vi "Shared Variable RT Driver VI.vi"(7 "Operation":T1, 11 "Device Reference in":T2 format="%.0x") -> (0 "Error Code":i32)   [LabVIEW 2015, in "Shared Variable Custom Device.lvlib"]
uses:
  Shared Variable Custom Device.lvlib
  <vilib>/NI Veristand/Custom Device API/Custom Device Item Ref.ctl
  <vilib>/NI Veristand/Custom Device API/Hardware Interface Driver VI Operation.ctl
  Support/HW Inline Ctrl.ctl
  <vilib>/NI Veristand/Custom Device API/Block Data Reference.ctl
  <vilib>/NI Veristand/Custom Device API/Data Reference.ctl
  Async/Input Data Control.ctl
  <vilib>/Utility/VariantDataType/Type.ctl
  <vilib>/NI Veristand/Custom Device API/Custom Device API.lvlib
  <vilib>/Utility/VariantDataType/VariantType.lvlib
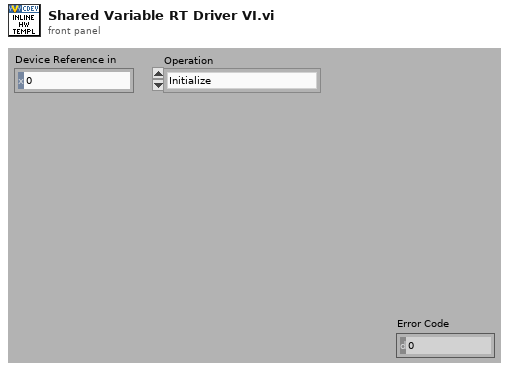
[diagram p1: front panel]
types:
  T1 = typedef "Custom Device API.lvlib/Hardware Interface Driver VI Operation.ctl" = enum16{"Initialize", "Start", "Read Data from HW", "Write Data to HW", "Close"}
  T2 = typedef "Custom Device API.lvlib/Custom Device Item Ref.ctl" = u64
  T3 = typedef "Shared Variable Custom Device.lvlib/HW Inline Ctrl.ctl" = cluster{"Status Notifier":refnum<notifier>, "RT FIFO Read":refnum<k33>, "RT FIFO Write":refnum<k33>, "Input Channels":cluster{"Input Values":dbl[], "Input Block Data Refs":T4[]}, "Output Channels":cluster{"Output Values":dbl[], "Output Block Data Refs":T4[]}, "error":errorcluster, "Timeout":i32, "Device Name":string}
  T4 = typedef "Custom Device API.lvlib/Block Data Reference.ctl" = cluster{"Data Reference":T5, "Offset":u64, "Length":u64}
  T5 = typedef "Custom Device API.lvlib/Data Reference.ctl" = i32
  T6 = typedef "Shared Variable Custom Device.lvlib/Input Data Control.ctl" = cluster{"Status Notifier":refnum<notifier>, "RT FIFO Read Cluster":cluster{"Read Values":dbl[], "Read Shared Variable Array":string[], "Read Channel Type Array":T7[]}, "RT FIFO Write Cluster":cluster{"Write Values":dbl[], "Write Shared Variable Array":string[], "Write Channel Type Array":T7[]}, "RT FIFO Read":refnum<k33>, "RT FIFO Write":refnum<k33>, "Device Name":string}
  T7 = typedef "VariantType.lvlib/Type.ctl" = enum8{"Invalid Type", "Void", "I8", "I16", "I32", "I64", "U8", "U16", "U32", "U64", "Single Float", "Double Float", "Extended Float", "Single Complex", "Double Complex", "Extended Complex", "Enum U8", "Enum U16", "Enum U32", "Enum U64", "Single Float With Unit", "Double Float With Unit", "Extended Float With Unit", "Single Complex with Unit", "Double Complex with Unit", "Extended Complex with Unit", "Boolean", "String", "Path", "Picture", "Tag", "Array", "Cluster", "Variant", "LV Variant", "Waveform", "Timestamp", "Digital Waveform", "Digital Data", "ExpressData", "Refnum", "External Data", "VI", "Poly VI", "LabVIEW Class Instance", "Fixed Point"}
  T8 = typedef "Shared Variable Custom Device.lvlib/Channel Information Control.ctl" = cluster{"Channel Refs":T2[], "Shared Variable URL Array":string[], "Channel Type Array":T7[], "Channel Type Glyph Array":i32[]}
  T9 = cluster{"Output Values":dbl[], "Output Block Data Refs":T4[]}
  T10 = cluster{"Input Values":dbl[], "Input Block Data Refs":T4[]}
  T11 = typedef "Custom Device API.lvlib/Custom Device Item Info.ctl" = cluster{"Name":string, "Is Channel":bool, "GUID":string, "Is Waveform":bool}
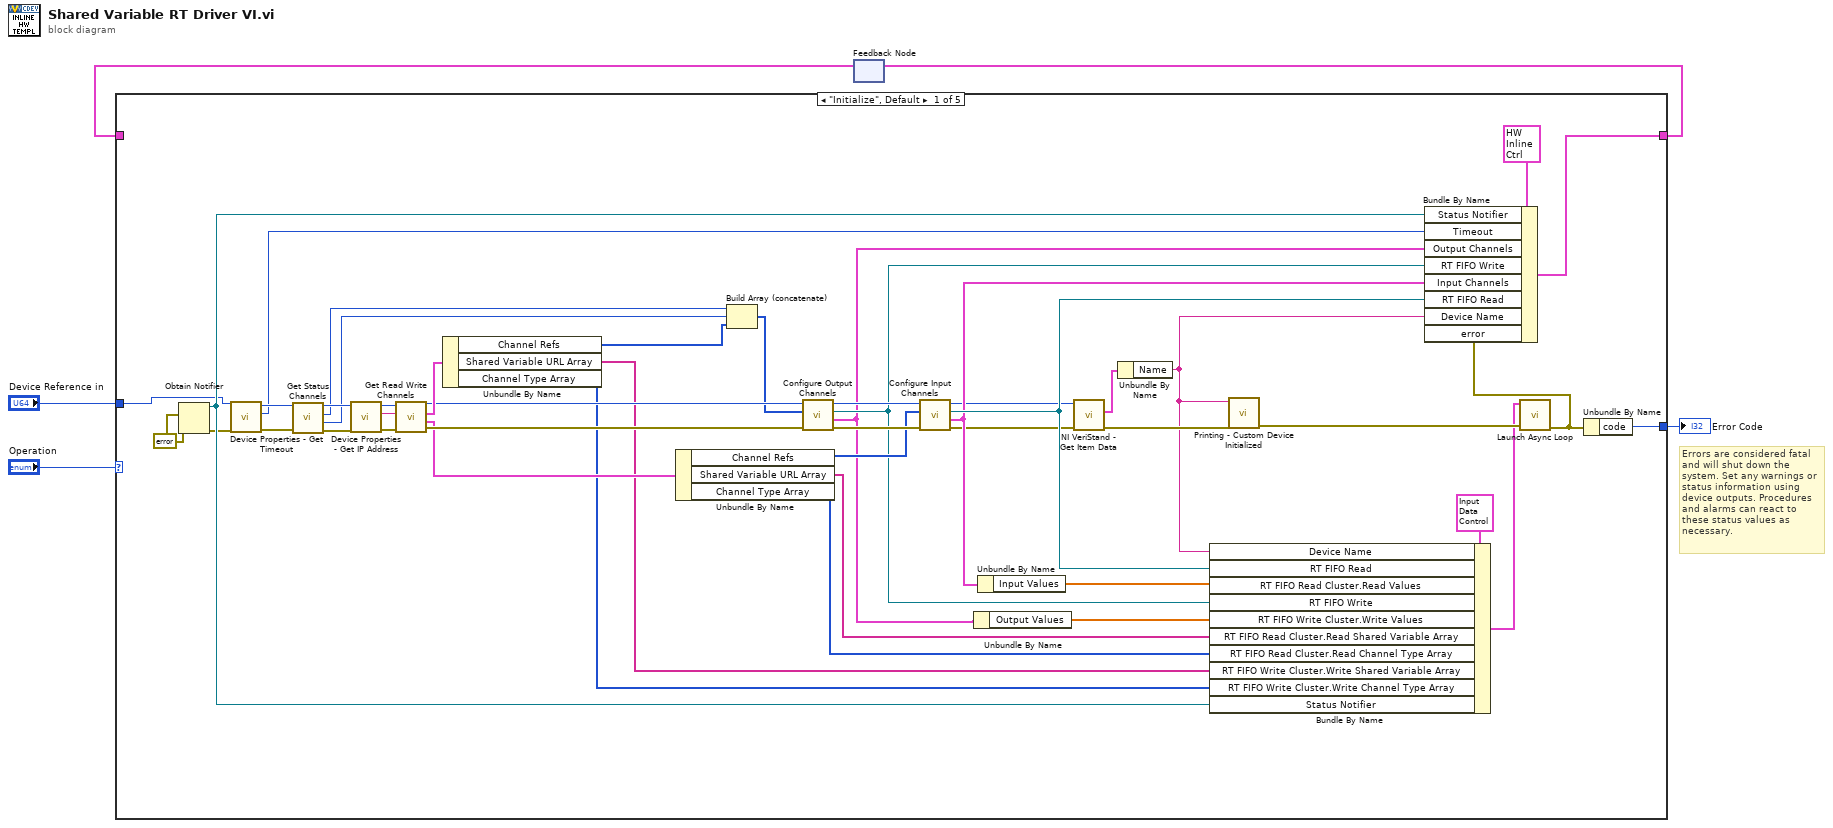
[diagram p0: block diagram]
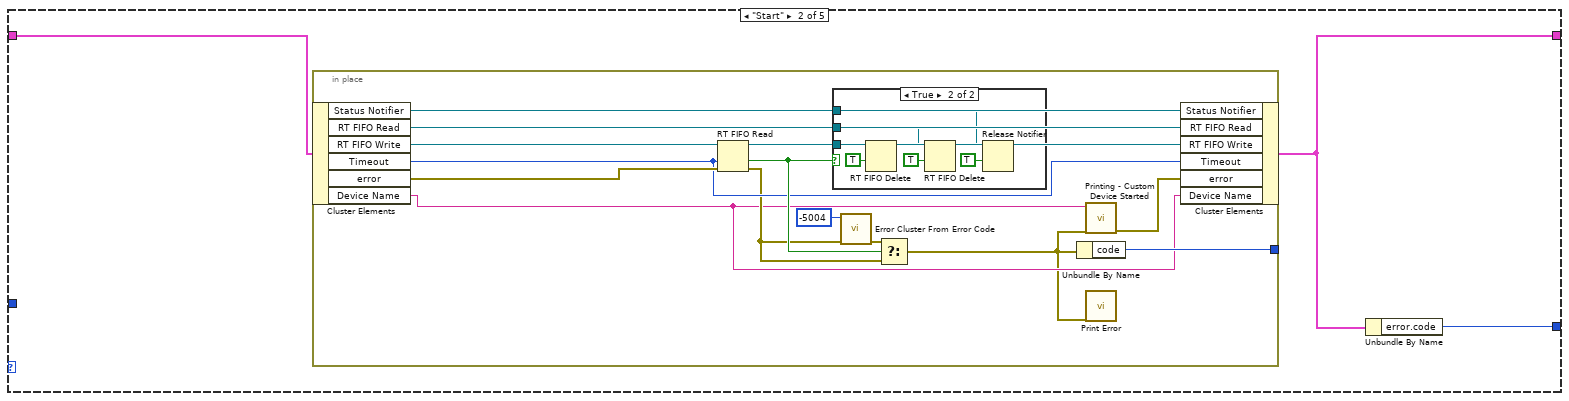
[diagram p2: hidden frame]
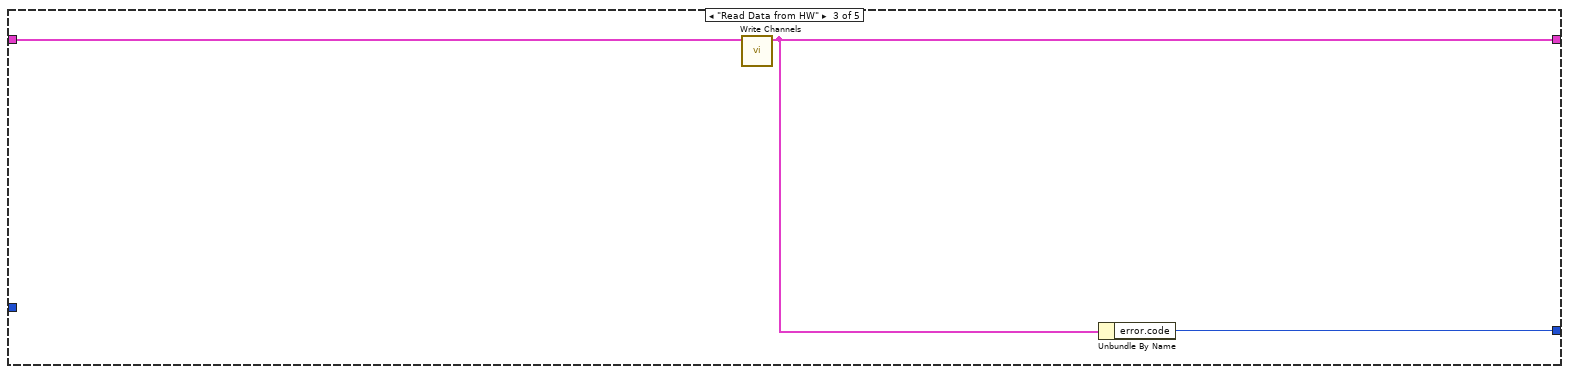
[diagram p4: hidden frame]
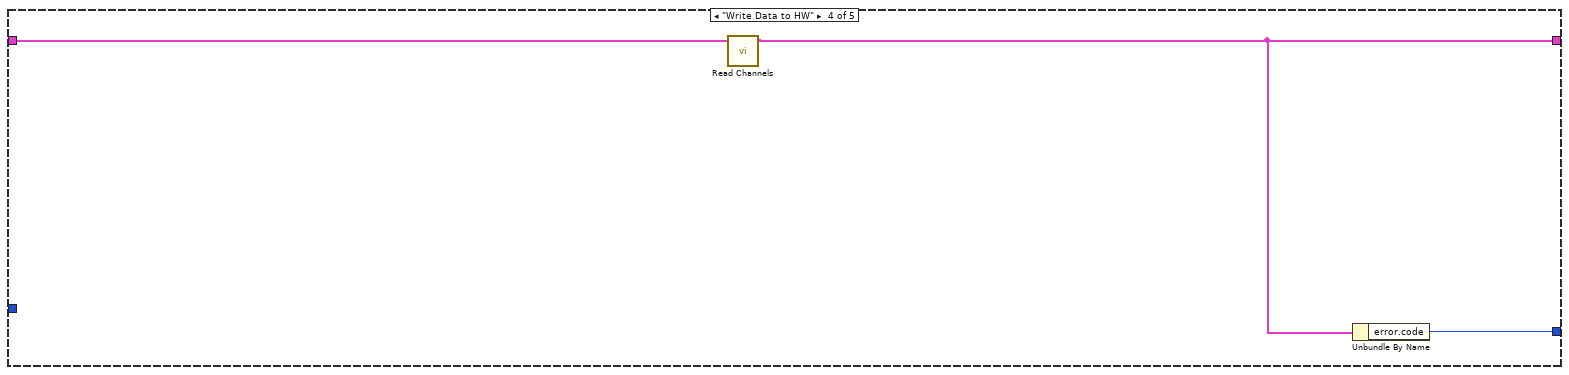
[diagram p5: hidden frame]
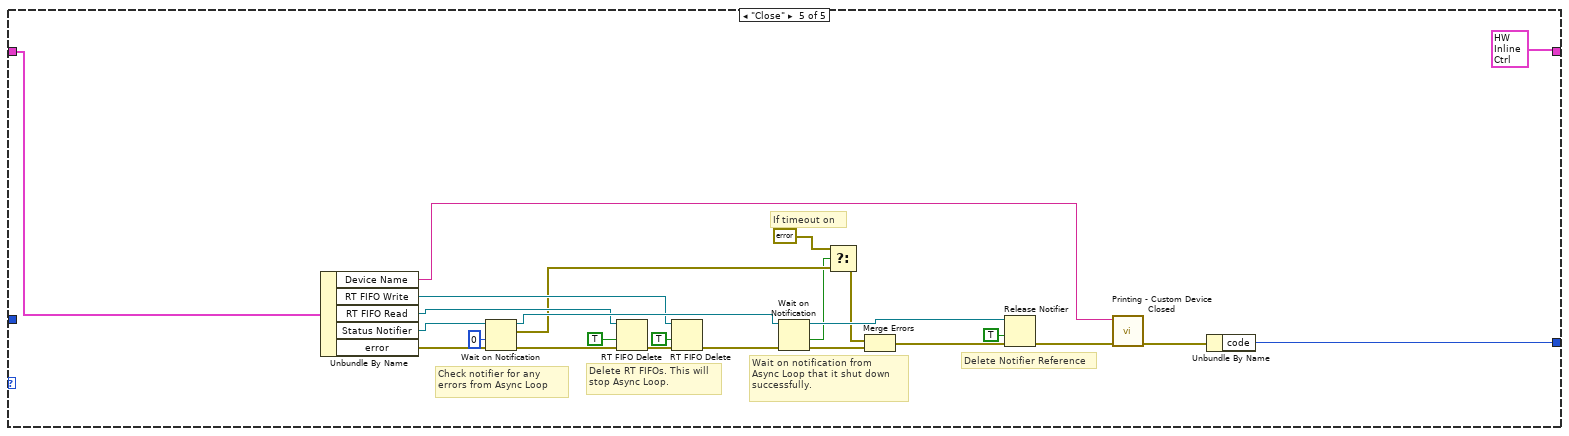
[diagram p6: hidden frame]
diagram:
  # "Errors are considered fatal and will shut down the system. Set any warnings or status information using device outputs. Procedures and alarms can react to these status values as necessary."
  n1 = feedback #1() -> (w3:T3)  [unwired: 1 out]
  n2 = case shown="\"Initialize\", Default" "Operation" {
    tunnel: [w48 w51 w75 w78 T3 {"Status Notifier"=refnum, "RT FIFO Read"=refnum, "RT FIFO Write"=refnum, "Input Channels"={"Input Values"=[], "Input Block Data Refs"=[]}, "Output Channels"={"Output Values"=[], "Output Block Data Refs"=[]}, "error"={"status"=FALSE, "code"=0, "source"=""}, "Timeout"=0, "Device Name"=""} ("HW Inline Ctrl out")] -> w4
    tunnel: w3 -> [_ w52 w76 w79 w81]
    tunnel: "Device Reference in" -> [w15 _ _ _ _]
    tunnel: [w50 w53 w74 w77 w104] -> w1
    frame "Initialize", Default {
      w47 = errorcluster {"status"=FALSE, "code"=0, "source"=""} ("error in (no error)")
      n3 = Obtain Notifier(notification data type=w47, error in (no error)=w47) -> (notifier out=w17:refnum<notifier>, error out=w14:errorcluster)  [unwired: 2 in, 1 out]
      n4 = call "Device Properties - Get Timeout.vi"("error in (no error)"=w14, "Device Ref in"=w15) -> ("error out"=w23:errorcluster, "IP Address"=w21:i32, "Device Ref out"=w22:T2)  [unwired: 7 in]
      n5 = call "Get Status Channels.vi"("error in (no error)"=w23, "Device Ref in"=w22) -> ("error out"=w46:errorcluster, "Error Code Ref"=w40:T2, "Connection Status Ref"=w41:T2, "Device Ref out"=w45:T2)  [unwired: 6 in]
      n6 = call "Device Properties - Get IP Address.vi"("error in (no error)"=w46, "Device Ref in"=w45) -> ("error out"=w42:errorcluster, "IP Address"=w43:string, "Device Ref out"=w44:T2)  [unwired: 7 in]
      n7 = call "Get Read Write Channels.vi"("error in (no error)"=w42, "IP Address"=w43, "Device Ref in"=w44) -> ("error out"=w39:errorcluster, "Input Channel Refs"=w32:T8, "Output Channel Refs"=w38:T8, "Device Ref out"=w37:T2)  [unwired: 5 in]
      n8 = Unbundle By Name(w38) -> ("Channel Refs"=w36:T2[], "Shared Variable URL Array"=w7:string[], "Channel Type Array"=w19:T7[])
      n9 = Unbundle By Name(w32) -> ("Channel Refs"=w31:T2[], "Shared Variable URL Array"=w8:string[], "Channel Type Array"=w20:T7[])
      n10 = Build Array (concatenate)(w41, w40, w36) -> (w35:T2[])
      n11 = call "Configure Output Channels.vi"("error in (no error)"=w39, "Output Channel Refs"=w35, "Device Ref in"=w37) -> ("error out"=w34:errorcluster, "Output Channels"=w24:T9, "RT FIFO Write out"=w26:refnum<k33>, "Device Ref out"=w33:T2)  [unwired: 5 in]
      n12 = call "Configure Input Channels.vi"("error in (no error)"=w34, "Input Channel Refs"=w31, "Device Ref in"=w33) -> ("error out"=w13:errorcluster, "Input Channels"=w28:T10, "RT FIFO Read out"=w29:refnum<k33>, "Device Ref out"=w12:T2)  [unwired: 5 in]
      n13 = Unbundle By Name(w24) -> ("Output Values"=w25:dbl[])
      n14 = Unbundle By Name(w28) -> ("Input Values"=w27:dbl[])
      n15 = call <vilib>:"NI VeriStand - Get Item Data.vi"("error in (no error)"=w13, "Item Ref in"=w12) -> ("error out"=w11:errorcluster, "Item Info"=w18:T11)  [unwired: 6 in, 2 out]
      n16 = Unbundle By Name(w18) -> ("Name"=w9:string)
      n17 = Bundle By Name(cluster=T6 {"Status Notifier"=refnum, "RT FIFO Read Cluster"={"Read Values"=[], "Read Shared Variable Array"=[], "Read Channel Type Array"=[]}, "RT FIFO Write Cluster"={"Write Values"=[], "Write Shared Variable Array"=[], "Write Channel Type Array"=[]}, "RT FIFO Read"=refnum, "RT FIFO Write"=refnum, "Device Name"=""} ("Input Data"), "Device Name"=w9, "RT FIFO Read"=w29, "RT FIFO Read Cluster.Read Values"=w27, "RT FIFO Write"=w26, "RT FIFO Write Cluster.Write Values"=w25, "RT FIFO Read Cluster.Read Shared Variable Array"=w8, "RT FIFO Read Cluster.Read Channel Type Array"=w20, "RT FIFO Write Cluster.Write Shared Variable Array"=w7, "RT FIFO Write Cluster.Write Channel Type Array"=w19, "Status Notifier"=w17) -> (w6:T6)
      n18 = call "Printing - Custom Device Initialized.vi"("error in (no error)"=w11, "Name"=w9) -> ("error out"=w10:errorcluster)  [unwired: 9 in]
      n19 = call "Launch Async Loop.vi"("error in (no error)"=w10, "Input Data"=w6) -> ("error out"=w16:errorcluster)  [unwired: 9 in]
      n20 = Bundle By Name(cluster=T3 {"Status Notifier"=refnum, "RT FIFO Read"=refnum, "RT FIFO Write"=refnum, "Input Channels"={"Input Values"=[], "Input Block Data Refs"=[]}, "Output Channels"={"Output Values"=[], "Output Block Data Refs"=[]}, "error"={"status"=FALSE, "code"=0, "source"=""}, "Timeout"=0, "Device Name"=""} ("HW Inline Ctrl"), "Status Notifier"=w17, "Timeout"=w21, "Output Channels"=w24, "RT FIFO Write"=w26, "Input Channels"=w28, "RT FIFO Read"=w29, "Device Name"=w9, "error"=w16) -> (w48:T3)
      n21 = Unbundle By Name(w16) -> ("code"=w50:i32)
    }
    frame "Start" {
      n22 = in-place {
        in-place-border: [w65] -> _
        n23 = in-place-cluster #2(w52) -> ("Status Notifier"=w59:refnum<notifier>, "RT FIFO Read"=w61:refnum<k33>, "RT FIFO Write"=w67:refnum<k33>, "Timeout"=w58:i32, "error"=w66:errorcluster, "Device Name"=w56:string)
        n24 = RT FIFO Read(0:w67, 2:w58, 3:w66) -> (8:w60:refnum<k33>, 10:w62:bool, 11:w57:errorcluster)  [unwired: 1 in, 2 out]
        n25 = case shown="True" w62 {
          tunnel: w60 -> [_ w72]
          tunnel: w61 -> [_ w73]
          tunnel: w59 -> [_ w69]
          frame False {
          }
          frame True {
            n26 = RT FIFO Delete(0:w72, 2:TRUE ("force destroy? (F)")) -> ()  [unwired: 1 in, 1 out]
            n27 = RT FIFO Delete(0:w73, 2:TRUE ("force destroy? (F)")) -> ()  [unwired: 1 in, 1 out]
            n28 = Release Notifier(notifier=w69, force destroy? (F)=TRUE) -> ()  [unwired: 1 in, 3 out]
          }
        }
        n29 = call <vilib>:"Error Cluster From Error Code.vi"("error in (no error)"=w57, "error code (0)"=-5004) -> ("error out"=w64:errorcluster)  [unwired: 7 in]
        n30 = Select(t=w64, s=w62, f=w57) -> (s? t:f=w54:errorcluster)
        n31 = Unbundle By Name(w54) -> ("code"=w65:i32)
        n32 = call "Printing - Custom Device Started.vi"("error in (no error)"=w54, "Name"=w56) -> ("error out"=w55:errorcluster)  [unwired: 9 in]
        n33 = call "Print Error.vi"("error in (no error)"=w54) -> ()  [unwired: 11 in]
        n34 = in-place-cluster #2("Status Notifier"=w59, "RT FIFO Read"=w61, "RT FIFO Write"=w60, "Timeout"=w58, "error"=w55, "Device Name"=w56) -> (w51:T3)
      }
      n35 = Unbundle By Name(w51) -> ("error.code"=w53:i32)
    }
    frame "Read Data from HW" {
      n36 = call "Write Channels.vi"("HW Inline Ctrl in"=w76) -> ("HW Inline Ctrl out"=w75:T3)  [unwired: 10 in]
      n37 = Unbundle By Name(w75) -> ("error.code"=w74:i32)
    }
    frame "Write Data to HW" {
      n38 = call "Read Channels.vi"("HW Inline Ctrl in"=w79) -> ("HW Inline Ctrl out"=w78:T3)  [unwired: 10 in]
      n39 = Unbundle By Name(w78) -> ("error.code"=w77:i32)
    }
    frame "Close" {
      # "Delete Notifier Reference"
      # "Wait on notification from\nAsync Loop that it shut down\nsuccessfully."
      # "Delete RT FIFOs. This will\nstop Async Loop."
      # "Check notifier for any\nerrors from Async Loop"
      # "If timeout on"
      n40 = Unbundle By Name(w81) -> ("Device Name"=w82:string, "RT FIFO Write"=w93:refnum<k33>, "RT FIFO Read"=w92:refnum<k33>, "Status Notifier"=w94:refnum<notifier>, "error"=w91:errorcluster)
      n41 = Wait on Notification(notifier=w94, timeout in ms (-1)=0, error in (no error)=w91) -> (notifier out=w96:refnum<notifier>, notification=w89:errorcluster, error out=w97:errorcluster)  [unwired: 1 in, 1 out]
      n42 = RT FIFO Delete(0:w92, 2:TRUE ("force destroy? (F)"), 3:w97) -> (11:w102:errorcluster)
      n43 = RT FIFO Delete(0:w93, 2:TRUE ("force destroy? (F)"), 3:w102) -> (11:w87:errorcluster)
      n44 = Wait on Notification(notifier=w96, error in (no error)=w87) -> (notifier out=w95:refnum<notifier>, timed out?=w88:bool, error out=w85:errorcluster)  [unwired: 2 in, 1 out]
      n45 = Select(t=errorcluster {"status"=FALSE, "code"=-5005, "source"=""}, s=w88, f=w89) -> (s? t:f=w86:errorcluster)
      n46 = Merge Errors(w86, w85) -> (w84:errorcluster)
      n47 = Release Notifier(notifier=w95, force destroy? (F)=TRUE, error in (no error)=w84) -> (error out=w83:errorcluster)  [unwired: 2 out]
      n48 = call "Printing - Custom Device Closed.vi"("error in (no error)"=w83, "Name"=w82) -> ("error out"=w80:errorcluster)  [unwired: 9 in]
      n49 = Unbundle By Name(w80) -> ("code"=w104:i32)
    }
  }
  "Error Code" <- w1
  n50 = feedback-in #1(w4) -> ()
